vi "Automated V&V Tx Rx.vi"() -> ()   [LabVIEW 2012, in "UART_Host_Driver.lvlib" / "UART Driver.lvclass"]
doc: "This example calls the UART Initialize, UART Configure Port, UART Execute Command, and a UART Close."
uses:
  UART Driver.lvclass
  FPGA/UART/StopBits.ctl
  FPGA/UART/Parity.ctl
  Typedefs/Configuration Parameters.ctl
  FPGA/UART/UART_Firmware.lvlib
  UART_Host_Driver.lvlib
panel:
  out "Failed Results Container":T3(array[cluster])
  out "Current Stop Bits( max 1)":i32
  out "Current Parity (max 2)":i32
  out "Passed Results Container":T3(array[cluster])
  out "Current Baud Iteration (max 13)":i32
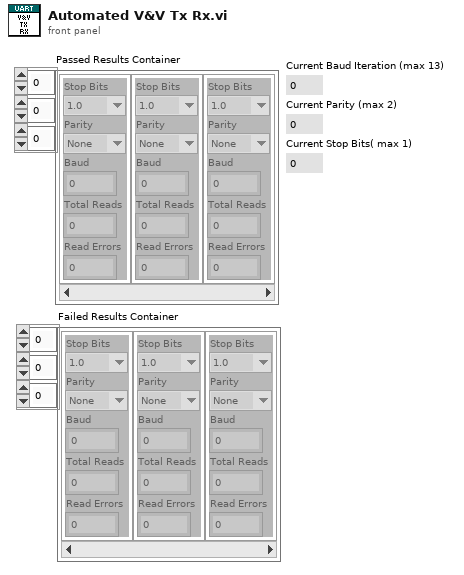
[diagram p1: front panel]
types:
  T1 = typedef "UART_Firmware.lvlib/StopBits.ctl" = enum8{"1.0", "1.5", "2.0"}
  T2 = typedef "UART_Firmware.lvlib/Parity.ctl" = enum8{"None", "Even", "Odd"}
  T3 = cluster{"Stop Bits":T1, "Parity":T2, "Baud":u32, "Total Reads":i32, "Read Errors":i32}[][][]
  T4 = enum16{"open", "replace", "create", "open or create", "replace or create", "replace or create with confirmation"}
  T5 = cluster{"Stop Bits":T1, "Parity":T2, "Baud":u32, "Total Reads":i32, "Read Errors":i32}
  T6 = typedef "UART_Host_Driver.lvlib/Configuration Parameters.ctl" = cluster{"Baud":u32, "Character Length":u8, "Stop Bits":T1, "Parity":T2, "Character Spacing (ticks)":u32}
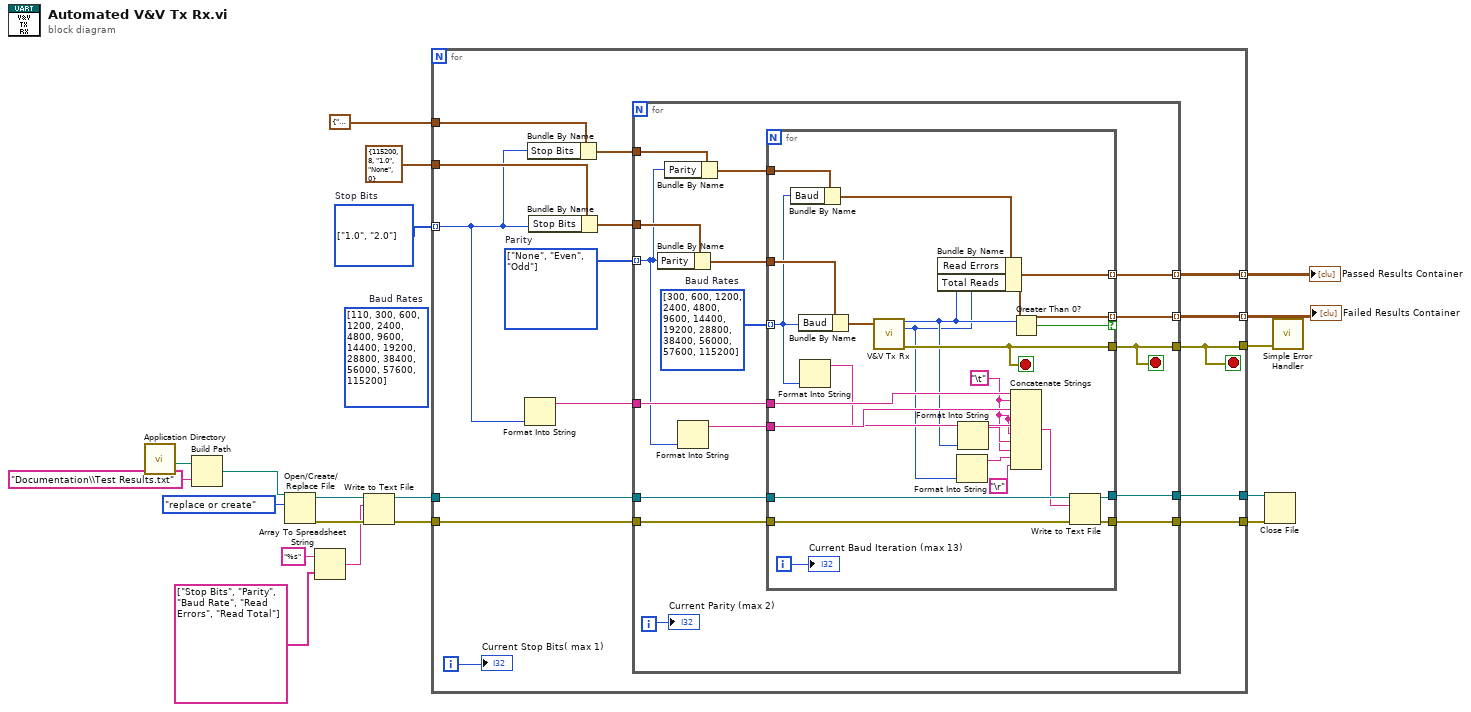
[diagram p0: block diagram]
diagram:
  (unwired) u32[] [110, 300, 600, 1200, 2400, 4800, 9600, 14400, 19200, 28800, 38400, 56000, 57600, 115200]  # Baud Rates
  w19 = T1[] [enum."1.0", enum."2.0"] items=["1.0", "1.5", "2.0"]  # Stop Bits
  n1 = call <vilib>:"Application Directory.vi"() -> ("Application Directory"=w3:path)
  n2 = Build Path(base path=w3, name or relative path="Documentation\\Test Results.txt") -> (appended path=w1:path)
  n3 = Open/Create/Replace File(file path (use dialog)=w1, operation (0:open)=T4."replace or create") -> (refnum out=w10:refnum<file>, error out=w9:errorcluster)  [unwired: 4 in, 1 out]
  n4 = Array To Spreadsheet String(array=string[] ["Stop Bits", "Parity", "Baud Rate", "Read Errors", "Read Total"], 3:"%s" ("format string")) -> (spreadsheet string=w5:string)  [unwired: 1 in]
  n5 = Write to Text File(file (use dialog)=w10, text=w5, error in=w9) -> (refnum out=w7:refnum<file>, error out=w8:errorcluster)  [unwired: 1 in, 1 out]
  n6 = for {
    tunnel: w19 -> [w25] mode=indexing
    tunnel: T6 {"Baud"=115200, "Character Length"=8, "Stop Bits"=enum."1.0", "Parity"=enum."None", "Character Spacing (ticks)"=0} ("Configuration Parameters") -> [w34]
    tunnel: [w26] -> w17
    tunnel: T5 {"Stop Bits"=enum."1.0", "Parity"=enum."None", "Baud"=0, "Total Reads"=0, "Read Errors"=0} ("Test Result") -> [w31]
    tunnel: [w29] -> w15 mode=indexing
    tunnel: [w27] -> w14 mode=indexing
    tunnel: w7 -> [w23]
    tunnel: w8 -> [w22]
    tunnel: [w21] -> w11
    tunnel: [w20] -> w12
    i -> [w28]
    stop <- w26 stop-if-true
    w32 = T2[] [enum."None", enum."Even", enum."Odd"] items=["None", "Even", "Odd"]  # Parity
    n7 = Format Into String(w25) -> (resulting string=w24:string)  [unwired: 3 in, 1 out]
    n8 = Bundle By Name(cluster=w31, "Stop Bits"=w25) -> (w30:T5)
    n9 = Bundle By Name(cluster=w34, "Stop Bits"=w25) -> (w33:T6)
    n10 = for {
      tunnel: w33 -> [w50]
      tunnel: w32 -> [w40] mode=indexing
      tunnel: [w43] -> w26
      tunnel: w30 -> [w48]
      tunnel: [w46] -> w29 mode=indexing
      tunnel: [w44] -> w27 mode=indexing
      tunnel: w24 -> [w41]
      tunnel: w23 -> [w39]
      tunnel: w22 -> [w37]
      tunnel: [w36] -> w21
      tunnel: [w35] -> w20
      i -> [w45]
      stop <- w43 stop-if-true
      w42 = u32[] [300, 600, 1200, 2400, 4800, 9600, 14400, 19200, 28800, 38400, 56000, 57600, 115200]  # Baud Rates
      n11 = Bundle By Name(cluster=w50, "Parity"=w40) -> (w49:T6)
      n12 = Bundle By Name(cluster=w48, "Parity"=w40) -> (w47:T5)
      n13 = Format Into String(w40) -> (resulting string=w38:string)  [unwired: 3 in, 1 out]
      n14 = for {
        tunnel: w42 -> [w62] mode=indexing
        tunnel: [w71] -> w43
        tunnel: w49 -> [w70]
        tunnel: w47 -> [w69]
        tunnel: [w67] -> w46 mode=indexing
        tunnel: [w67] -> w44 mode=indexing if=w66
        tunnel: w41 -> [w65]
        tunnel: w39 -> [w64]
        tunnel: w38 -> [w63]
        tunnel: w37 -> [w55]
        tunnel: [w54] -> w36
        tunnel: [w53] -> w35
        i -> [w72]
        stop <- w71 stop-if-true
        w52 = "\t"
        n15 = Bundle By Name(cluster=w69, "Baud"=w62) -> (w68:T5)
        n16 = Bundle By Name(cluster=w70, "Baud"=w62) -> (w73:T6)
        n17 = Format Into String(w62) -> (resulting string=w61:string)  [unwired: 3 in, 1 out]
        n18 = call "V&V Tx Rx.vi"("Configuration Parameters"=w73) -> ("Number of Read Errors"=w60:i32, "Number of Reads Executed"=w59:i32, "error out"=w71:errorcluster)  [unwired: 12 in]
        n19 = Bundle By Name(cluster=w68, "Read Errors"=w60, "Total Reads"=w59) -> (w67:T5)
        n20 = Format Into String(w59) -> (resulting string=w57:string)  [unwired: 3 in, 1 out]
        n21 = Format Into String(w60) -> (resulting string=w58:string)  [unwired: 3 in, 1 out]
        n22 = Greater Than 0?(x=w60) -> (x > 0?=w66:bool)
        n23 = Concatenate Strings(w65, w52, w63, w52, w61, w52, w58, w52, w57, "\r") -> (w56:string)
        n24 = Write to Text File(file (use dialog)=w64, text=w56, error in=w55) -> (refnum out=w53:refnum<file>, error out=w54:errorcluster)  [unwired: 1 in, 1 out]
        "Current Baud Iteration (max 13)" <- w72
      }
      "Current Parity (max 2)" <- w45
    }
    "Current Stop Bits( max 1)" <- w28
  }
  "Passed Results Container" <- w15
  "Failed Results Container" <- w14
  n25 = Close File(refnum=w12, error in=w11) -> ()  [unwired: 2 out]
  n26 = call <vilib>:"Simple Error Handler.vi"("error in (no error)"=w17) -> ()  [unwired: 4 in, 5 out]
